vi "DCSAnalysis.vi"(0 "# Detectors":u32=8, 2 "File path":string, 3 "Frame #":u32, 5 "rho":dbl[](array[numeric])=[2.5, 2.5, 2.5, 2.5, 2.5, 2.5, 2.5, 2.5, -1.0, -1.0, -1.0, -1.0], 7 "other settings":u32[](array[numeric])=[0, 0, 0, 0, 0, 0, 0, 0, 0, 0, 0, 0], 8 "avgBool":bool[][](array[boolean]), 9 "var values":dbl[](array[numeric])=[0.0, 0.0, 0.0, 0.0, -1.0, -1.0, -1.0, -1.0, -1.0, -1.0, -1.0, -1.0]) -> (20 "Flow in each detector":dbl[](array[numeric])=[-1.0, -1.0, -1.0, -1.0, -1.0, -1.0, -1.0, -1.0, -1.0, -1.0, -1.0, -1.0], 23 "Tau":T1(graph) caption="Relative changes of flow", 27 "End":bool)   [LabVIEW 2016]
uses:
  GTcode_v6_Michelle/dll.dll
panel:
  out "avgInt1x32":u32[](array[numeric])
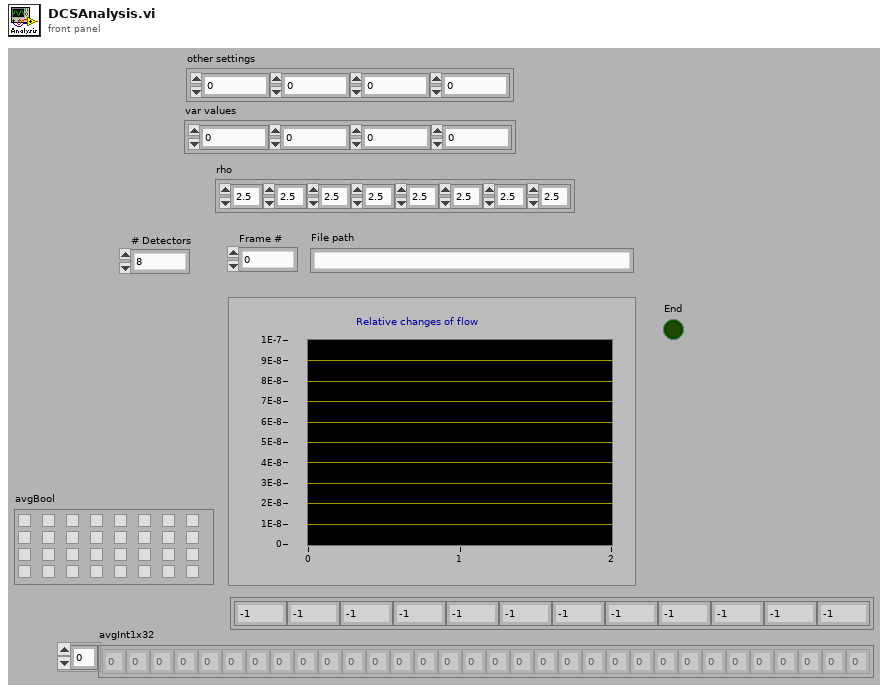
[diagram p1: front panel]
types:
  T1 = cluster{dbl, dbl, dbl, dbl, dbl, dbl, dbl, dbl, dbl, dbl, dbl, dbl}
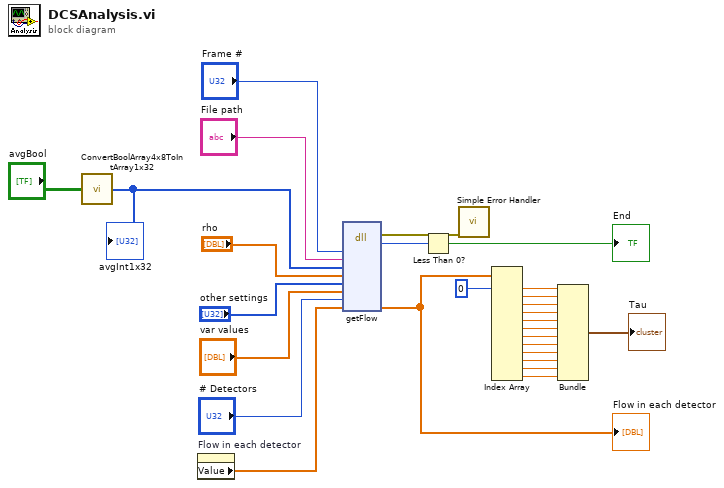
[diagram p0: block diagram]
diagram:
  n1 = call "ConvertBoolArray4x8ToIntArray1x32.vi"("boolMatrix4x8"="avgBool") -> ("intArray1x32"=w27:u32[])  [unwired: 14 in]
  "avgInt1x32" <- w27
  n2 = property on="Flow in each detector" class="Arr (strict)"() -> ("Value"=w21:dbl[])  [unwired: 2 in, 2 out]
  n3 = dll-call lib="C:/Users/BUCKLEY-ADMIN/Desktop/GTcode_v6_Michelle/dll.dll" fn="getFlow"("iFileIndex"="Frame #", "fileName"="File path", "avg"=w27, "rho"="rho", "set"="other settings", "var"="var values", "iDetectorCount"="# Detectors", "flow"=w21) -> (error out=w4:errorcluster, "return type"=w20:i32, "flow"=w24:dbl[])  [unwired: 10 in, 1 out]
  "Flow in each detector" <- w24
  n4 = Less Than 0?(x=w20) -> (x < 0?=→"End":bool)
  n5 = call <vilib>:"Simple Error Handler.vi"("error in (no error)"=w4) -> ()  [unwired: 4 in, 5 out]
  n6 = Index Array(array=w24, index #1=0) -> (element #1=w19:dbl, element #2=w18:dbl, element #3=w17:dbl, element #4=w16:dbl, element #5=w15:dbl, element #6=w14:dbl, element #7=w13:dbl, element #8=w12:dbl, element #9=w9:dbl, element #10=w8:dbl, element #11=w7:dbl, element #12=w6:dbl)  [unwired: 11 in]
  n7 = Bundle(w19, w18, w17, w16, w15, w14, w13, w12, w9, w8, w7, w6) -> (→"Tau":T1)  [unwired: 1 in]
